vi "SetTrack.vi"   [LabVIEW 2011]
uses:
  Robot Global Data.vi
types:
  T1 = typedef "WPI_JoystickDevRef.ctl" = cluster{"Device":T2}
  T2 = typedef "WPI_JoystickDeviceEnum.ctl" = enum16{"USB 1", "USB 2", "USB 3", "USB 4", "Kinect 1", "Kinect 2"}
  T3 = typedef "WPI_JoystickButtonState.ctl" = cluster{"Button 1":bool, "Button 2":bool, "Button 3":bool, "Button 4":bool, "Button 5":bool, "Button 6":bool, "Button 7":bool, "Button 8":bool, "Button 9":bool, "Button 10":bool, "Button 11":bool, "Button 12":bool}
  T4 = cluster{"axis 1 (x)":dbl, "axis 2 (y)":dbl, "axis 3 (throttle)":dbl, "axis 4":dbl, "axis 5":dbl, "axis 6":dbl}
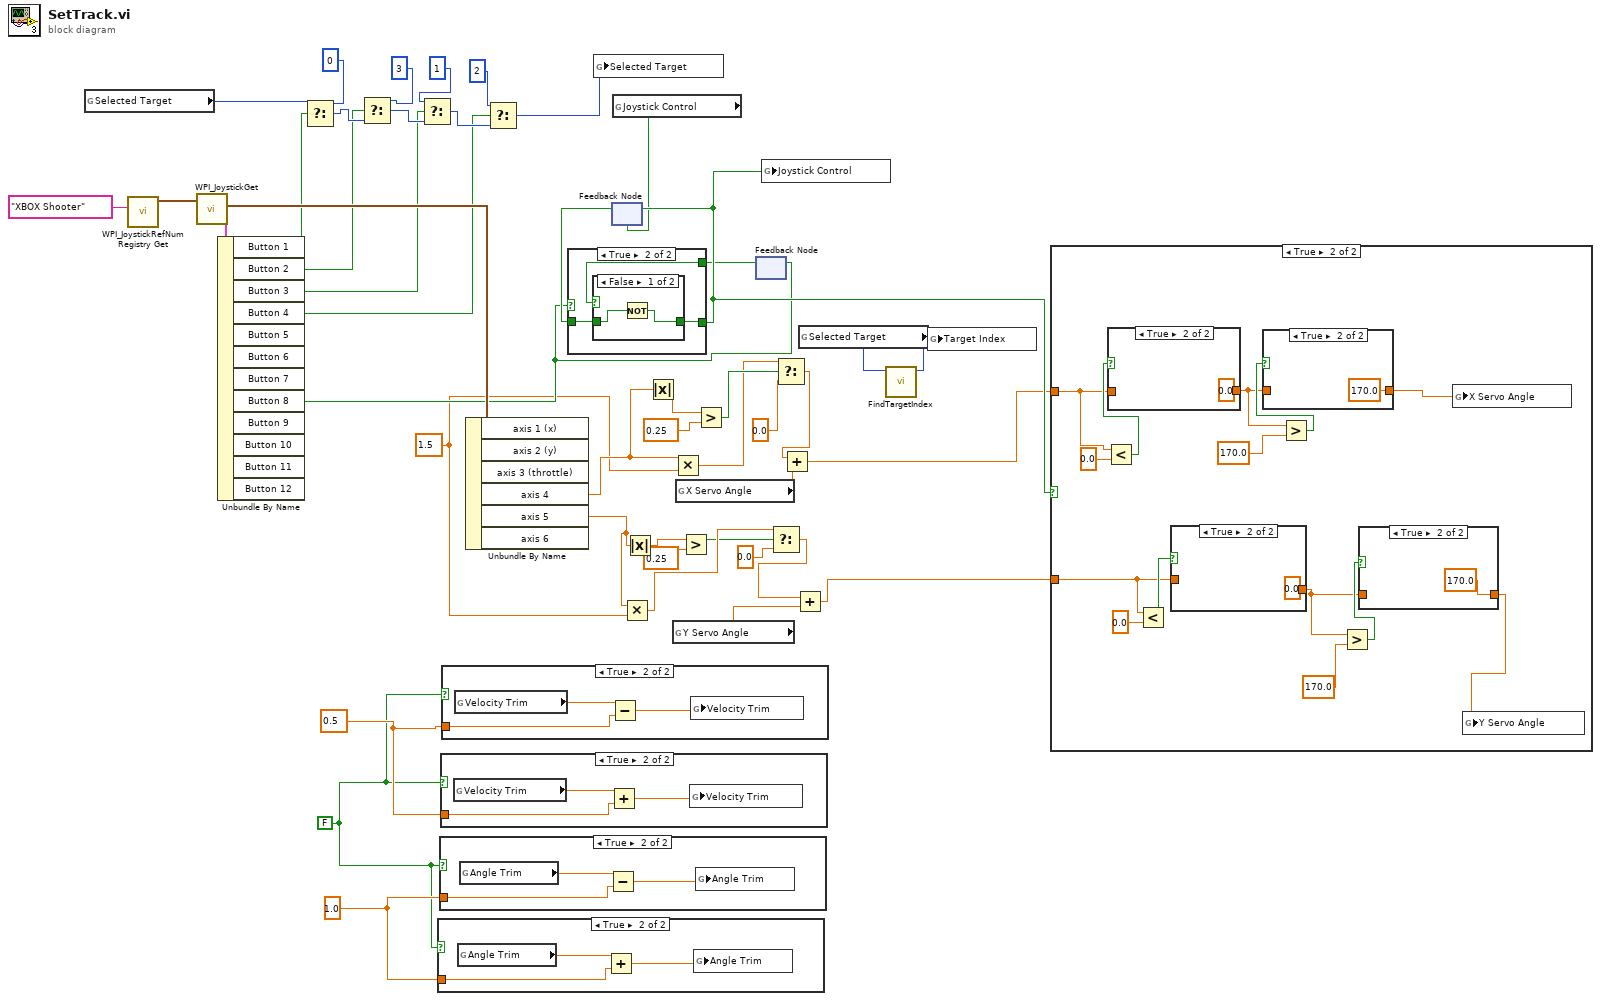
[diagram p0: block diagram]
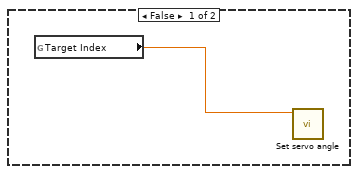
[diagram p8: hidden frame]
diagram:
  w1 = FALSE
  w2 = 1.0 ("y")
  w3 = 0.5 ("y")
  w4 = 1.5
  n1 = global read "Robot Global Data.vi" "Selected Target"() -> (w18:i32)
  n2 = call <vilib>:"WPI_JoystickRefNum Registry Get.vi"("refnum name"="XBOX Shooter") -> ("JoystickDevRef"=w41:T1)  [unwired: 9 in, 1 out]
  n3 = call <vilib>:"WPI_JoystickGet.vi"("JoystickDevRef"=w41) -> ("Buttons"=w46:T3, "Axes"=w45:T4)  [unwired: 4 in, 1 out]
  n4 = Unbundle By Name(w46) -> ("Button 1"=w19:bool, "Button 2"=w15:bool, "Button 3"=w12:bool, "Button 4"=w10:bool, "Button 8"=w21:bool)  [unwired: 7 out]
  n5 = Select(t=0, s=w19, f=w18) -> (s? t:f=w16:i32)
  n6 = Select(t=3, s=w15, f=w16) -> (s? t:f=w13:i32)
  n7 = Select(t=1, s=w12, f=w13) -> (s? t:f=w11:i32)
  n8 = case shown="True" w1 {
    tunnel: w2 -> [_ w47]
    frame False {
    }
    frame True {
      n9 = global read "Robot Global Data.vi" "Angle Trim"() -> (w49:dbl)
      n10 = Add(x=w49, y=w47) -> (x+y=w48:dbl)
      n11 = global write "Robot Global Data.vi" "Angle Trim"(w48) -> ()
    }
  }
  n12 = case shown="True" w1 {
    tunnel: w2 -> [_ w50]
    frame False {
    }
    frame True {
      n13 = global read "Robot Global Data.vi" "Angle Trim"() -> (w52:dbl)
      n14 = Subtract(x=w52, y=w50) -> (x-y=w51:dbl)
      n15 = global write "Robot Global Data.vi" "Angle Trim"(w51) -> ()
    }
  }
  n16 = case shown="True" w1 {
    tunnel: w3 -> [_ w53]
    frame False {
    }
    frame True {
      n17 = global read "Robot Global Data.vi" "Velocity Trim"() -> (w55:dbl)
      n18 = Add(x=w55, y=w53) -> (x+y=w54:dbl)
      n19 = global write "Robot Global Data.vi" "Velocity Trim"(w54) -> ()
    }
  }
  n20 = case shown="True" w1 {
    tunnel: w3 -> [_ w56]
    frame False {
    }
    frame True {
      n21 = global read "Robot Global Data.vi" "Velocity Trim"() -> (w58:dbl)
      n22 = Subtract(x=w58, y=w56) -> (x-y=w57:dbl)
      n23 = global write "Robot Global Data.vi" "Velocity Trim"(w57) -> ()
    }
  }
  n24 = Unbundle By Name(w45) -> ("axis 4"=w27:dbl, "axis 5"=w38:dbl)  [unwired: 4 out]
  n25 = Select(t=2, s=w10, f=w11) -> (s? t:f=w9:i32)
  n26 = global write "Robot Global Data.vi" "Selected Target"(w9) -> ()
  n27 = global read "Robot Global Data.vi" "Joystick Control"() -> (w20:bool)
  n28 = feedback #1(w20) -> (w43:bool)
  n29 = Multiply(x=w38, y=w4) -> (x*y=w37:dbl)
  n30 = Absolute Value(x=w38) -> (abs(x)=w36:dbl)
  n31 = Absolute Value(x=w27) -> (abs(x)=w31:dbl)
  n32 = Multiply(x=w27, y=w4) -> (x*y=w25:dbl)
  n33 = global read "Robot Global Data.vi" "Y Servo Angle"() -> (w40:dbl)
  n34 = global read "Robot Global Data.vi" "X Servo Angle"() -> (w23:dbl)
  n35 = Greater?(x=w36, y=0.25) -> (0:w34:bool)
  n36 = Greater?(x=w31, y=0.25) -> (0:w29:bool)
  n37 = feedback-in #2(w21) -> ()
  n38 = feedback #2() -> (w22:bool)  [unwired: 1 in]
  n39 = case shown="True" w21 {
    tunnel: w43 -> [w59 w62]
    tunnel: [w59 w61] -> w39
    tunnel: w22 -> [_ w60]
    frame False {
    }
    frame True {
      n40 = case shown="False" w60 {
        tunnel: w62 -> [w64 w65]
        tunnel: [w63 w65] -> w61
        frame False {
          n41 = Not(x=w64) -> (.not. x?=w63:bool)
        }
        frame True {
        }
      }
    }
  }
  n42 = feedback-in #1(w39) -> ()
  n43 = global write "Robot Global Data.vi" "Joystick Control"(w39) -> ()
  n44 = Select(t=w37, s=w34, f=0.0) -> (s? t:f=w32:dbl)
  n45 = Select(t=w25, s=w29, f=0.0) -> (s? t:f=w24:dbl)
  n46 = Add(x=w24, y=w23) -> (x+y=w26:dbl)
  n47 = Add(x=w32, y=w40) -> (x+y=w44:dbl)
  n48 = global read "Robot Global Data.vi" "Selected Target"() -> (w6:i32)
  n49 = call "FindTargetIndex.vi"("Selected Target"=w6) -> ("Target Index"=w5:i32)  [unwired: 10 in]
  n50 = global write "Robot Global Data.vi" "Target Index"(w5) -> ()
  n51 = case shown="True" w39 {
    tunnel: w44 -> [_ w77]
    tunnel: w26 -> [_ w67]
    frame False {
      n52 = global read "Robot Global Data.vi" "Target Index"() -> (w66:dbl)
      n53 = call "Set servo angle.vi"("Target Index"=w66) -> ()  [unwired: 11 in]
    }
    frame True {
      n54 = Less?(x=w67, y=0.0) -> (x < y?=w79:bool)
      n55 = case shown="True" w79 {
        tunnel: [w87 0.0] -> w69
        tunnel: w67 -> [w87 _]
        frame False {
        }
        frame True {
        }
      }
      n56 = Less?(x=w77, y=0.0) -> (x < y?=w78:bool)
      n57 = case shown="True" w78 {
        tunnel: w77 -> [w85 _]
        tunnel: [w85 0.0] -> w73
        frame False {
        }
        frame True {
        }
      }
      n58 = Greater?(x=w69, y=170.0) -> (0:w70:bool)
      n59 = case shown="True" w70 {
        tunnel: w69 -> [w81 _]
        tunnel: [w81 170.0] -> w71
        frame False {
        }
        frame True {
        }
      }
      n60 = Greater?(x=w73, y=170.0) -> (0:w74:bool)
      n61 = case shown="True" w74 {
        tunnel: w73 -> [w83 _]
        tunnel: [w83 170.0] -> w72
        frame False {
        }
        frame True {
        }
      }
      n62 = global write "Robot Global Data.vi" "X Servo Angle"(w71) -> ()
      n63 = global write "Robot Global Data.vi" "Y Servo Angle"(w72) -> ()
    }
  }
